vi "safedivide.vi"(10 "row_vec(sum)":dbl[](array[numeric]), 11 "V' x A":dbl[](array[numeric])) -> (3 "Array":dbl[](array[numeric]))   [LabVIEW 2014]
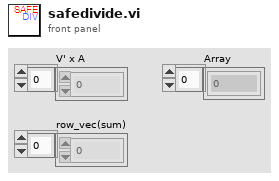
[diagram p1: front panel]
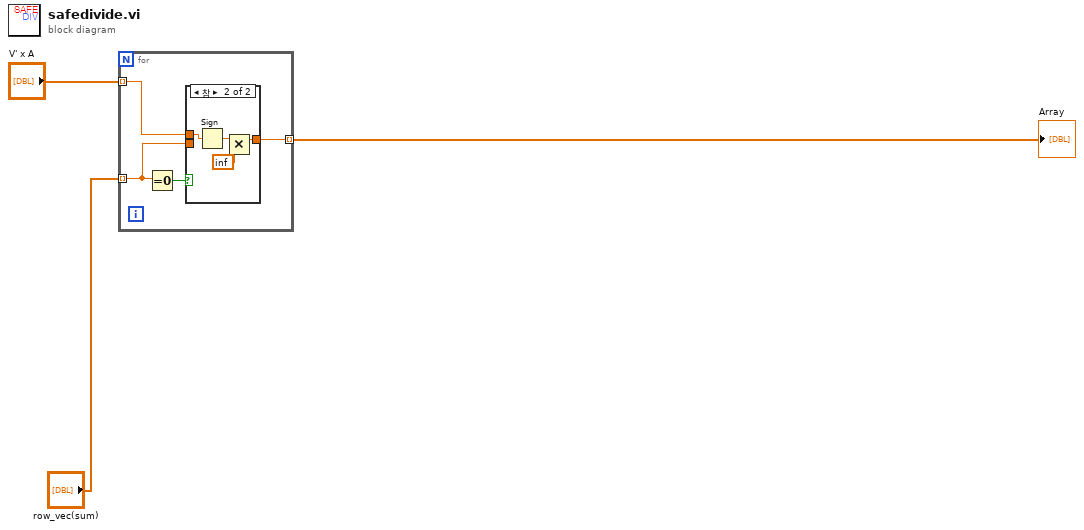
[diagram p0: block diagram]
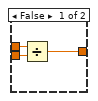
[diagram p2: hidden frame]
diagram:
  n1 = for {
    tunnel: "row_vec(sum)" -> [w5] mode=indexing
    tunnel: "V' x A" -> [w6] mode=indexing
    tunnel: [w4] -> w3 mode=indexing
    n2 = Equal To 0?(x=w5) -> (x = 0?=w7:bool)
    n3 = case shown="참" w7 {
      tunnel: w6 -> [w10 w11]
      tunnel: w5 -> [w9 _]
      tunnel: [w8 w13] -> w4
      frame False {
        n4 = Divide(x=w10, y=w9) -> (x/y=w8:dbl)
      }
      frame True {
        n5 = Sign(1:w11) -> (0:w12:dbl)
        n6 = Multiply(x=w12, y=inf) -> (x*y=w13:dbl)
      }
    }
  }
  "Array" <- w3
